vi "Flush File Data.vi"(8 "error in (no error)":errorcluster, 10 "File Log Spec in":T1={"Directory"=path "", "Groups"=[], "Buffer Size"=0, "Properties"=[], "Pretrigger"=FALSE, "Pretrigger Samples"=0, "Name"="", "Timestamp"=FALSE, "Error"=0, "Auto Open"=FALSE, "File Node Ref"=18446744073709551615, "Archive"=FALSE, "Archive Directory"=path "", "Segment Files"=FALSE, "Segment Files By"=enum."Size", "Segment Size"=100000, "Flushed Data Size Total"=0, "Append Waveform Properties"=FALSE, "Logging State"=enum."Not Started", "First Sample Start Time"=timestamp(0 s since 1904-01-01), "System dt"=0.0} {"File Node Ref" format="%.0x"}, 11 "TDMS File Ref in":refnum<k34>) -> (0 "error out":errorcluster, 2 "File Log Spec out":T1={"Directory"=path "", "Groups"=[], "Buffer Size"=0, "Properties"=[], "Pretrigger"=FALSE, "Pretrigger Samples"=0, "Name"="", "Timestamp"=FALSE, "Error"=0, "Auto Open"=FALSE, "File Node Ref"=18446744073709551615, "Archive"=FALSE, "Archive Directory"=path "", "Segment Files"=FALSE, "Segment Files By"=enum."Size", "Segment Size"=100000, "Flushed Data Size Total"=0, "Append Waveform Properties"=FALSE, "Logging State"=enum."Not Started", "First Sample Start Time"=timestamp(0 s since 1904-01-01), "System dt"=0.0} {"File Node Ref" format="%.0x"}, 3 "TDMS File Ref out":refnum<k34>)   [LabVIEW 2027, in "Embedded Data Logger Engine.lvlib"]
uses:
  Embedded Data Logger Engine.lvlib
  File Logging Specification.ctl
  Group Logging Specification.ctl
  Group Buffer Data.ctl
  Property Specification.ctl
  <vilib>/NI VeriStand/Custom Device API/Custom Device Item Ref.ctl
  Shared/Segment Files By.ctl
  Logging State.ctl
  Add to Flushed Data Size.vi
  <vilib>/NI VeriStand/Custom Device API/Custom Device API.lvlib
  Shared/Embedded Data Logger Shared.lvlib
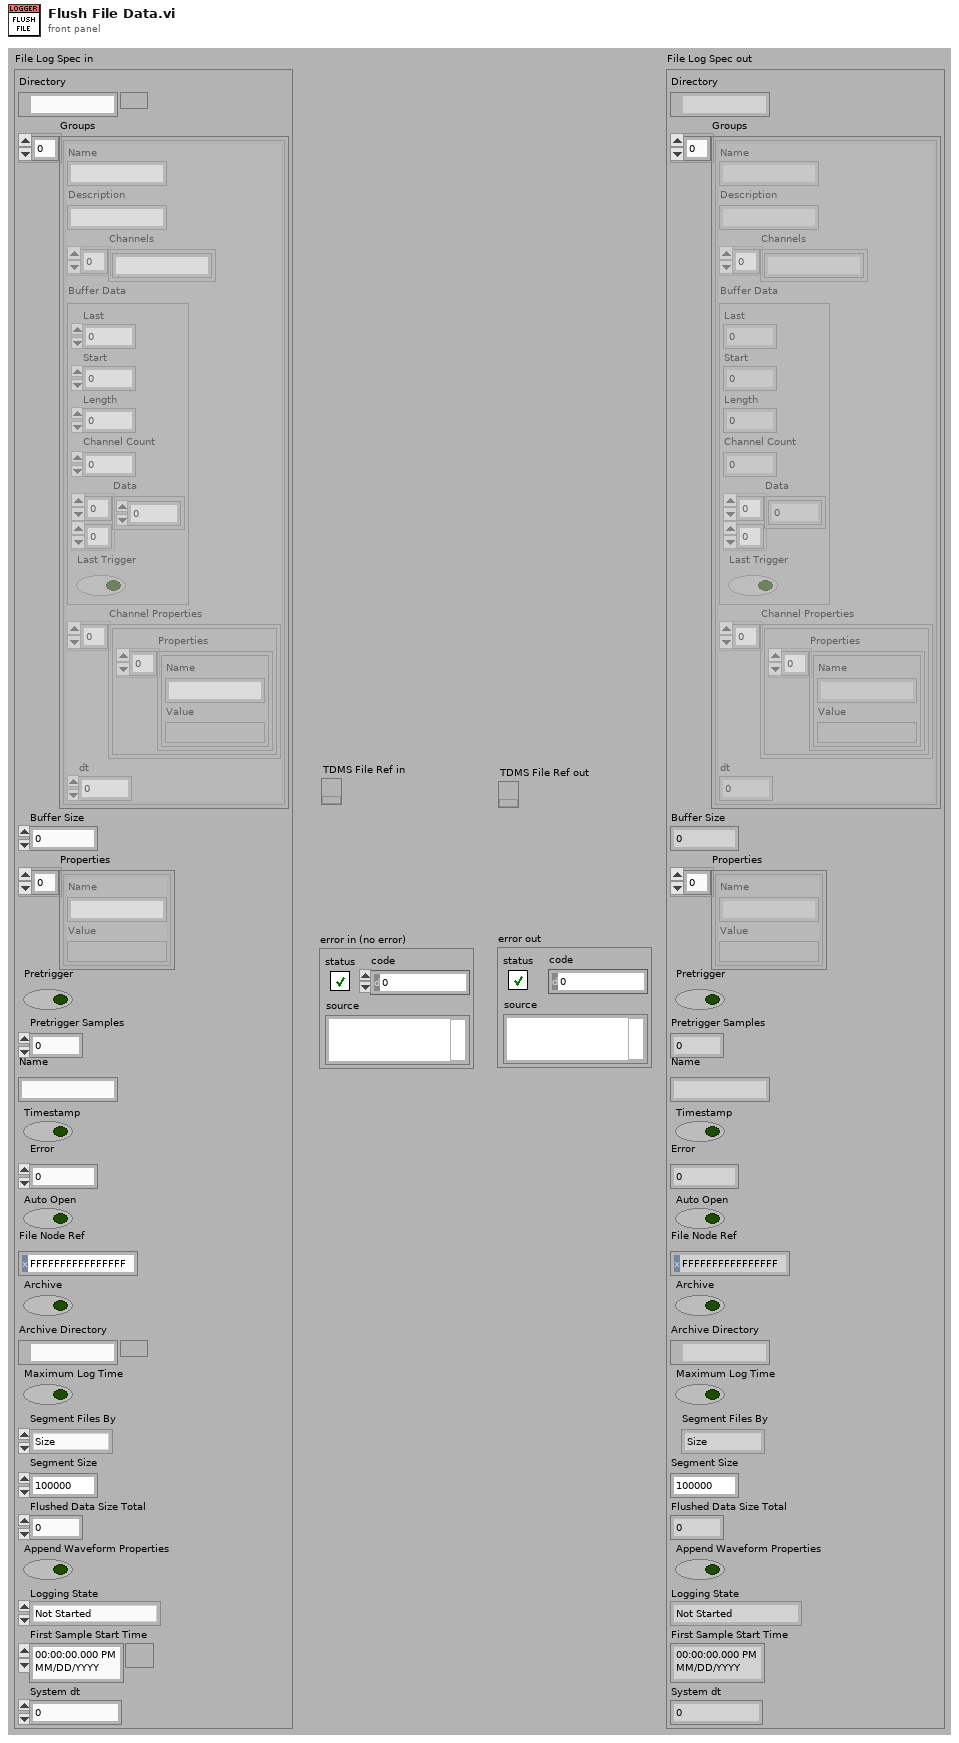
[diagram p1: front panel]
types:
  T1 = typedef "Embedded Data Logger Engine.lvlib/File Logging Specification.ctl" = cluster{"Directory":path, "Groups":T2[], "Buffer Size":i32, "Properties":T4[], "Pretrigger":bool, "Pretrigger Samples":i32, "Name":string, "Timestamp":bool, "Error":i32, "Auto Open":bool, "File Node Ref":T5, "Archive":bool, "Archive Directory":path, "Segment Files":bool, "Segment Files By":T6, "Segment Size":u32, "Flushed Data Size Total":u32, "Append Waveform Properties":bool, "Logging State":T7, "First Sample Start Time":timestamp, "System dt":dbl}
  T2 = typedef "Embedded Data Logger Engine.lvlib/Group Logging Specification.ctl" = cluster{"Name":string, "Description":string, "Channels":string[], "Buffer Data":T3, "Channel Properties":cluster{"Properties":T4[]}[], "dt":dbl}
  T3 = typedef "Embedded Data Logger Engine.lvlib/Group Buffer Data.ctl" = cluster{"Last":i32, "Start":i32, "Length":i32, "Channel Count":i32, "Data":dbl[][], "Last Trigger":bool}
  T4 = typedef "Embedded Data Logger Engine.lvlib/Property Specification.ctl" = cluster{"Name":string, "Value":variant}
  T5 = typedef "Custom Device API.lvlib/Custom Device Item Ref.ctl" = u64
  T6 = typedef "Embedded Data Logger Shared.lvlib/Segment Files By.ctl" = enum16{"Time", "Size"}
  T7 = typedef "Embedded Data Logger Engine.lvlib/Logging State.ctl" = enum16{"Not Started", "Continous Logging", "Paused", "Discontinous Logging"}
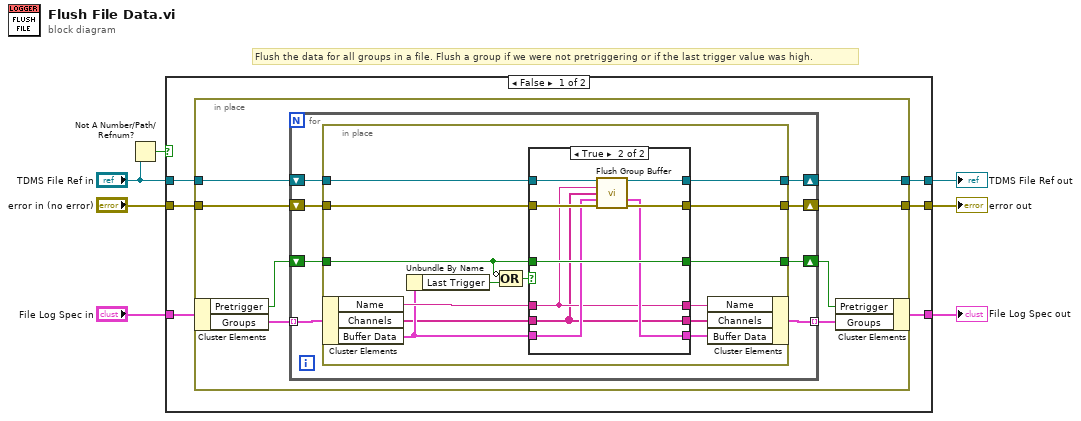
[diagram p0: block diagram]
diagram:
  # "Flush the data for all groups in a file. Flush a group if we were not pretriggering or if the last trigger value was high."
  n1 = Not A Number/Path/Refnum?(number/path/refnum="TDMS File Ref in") -> (NaN/Path/Refnum?=w1:bool)
  n2 = case shown="False" w1 {
    tunnel: "File Log Spec in" -> [w13 w59]
    tunnel: "TDMS File Ref in" -> [w12 w61]
    tunnel: [w11 w61] -> w5
    tunnel: [w10 w59] -> w7
    tunnel: "error in (no error)" -> [w9 w60]
    tunnel: [w8 w60] -> w6
    frame False {
      n3 = in-place {
        in-place-border: w12 -> [w21]
        in-place-border: [w20] -> w11
        in-place-border: w9 -> [w15]
        in-place-border: [w14] -> w8
        n4 = in-place-cluster #1(w13) -> ("Pretrigger"=w17:bool, "Groups"=w19:T2[])
        n5 = for {
          tunnel: w19 -> [w27] mode=indexing
          tunnel: [w26] -> w18 mode=indexing
          shift-right: [w28] -> w20
          shift-left: w21 -> [w29]
          shift-right: [w25] -> w16
          shift-left: w17 -> [w24]
          shift-right: [w22] -> w14
          shift-left: w15 -> [w23]
          n6 = in-place {
            in-place-border: w24 -> [w34]
            in-place-border: w29 -> [w38]
            in-place-border: [w39] -> w28
            in-place-border: [w33] -> w25
            in-place-border: w23 -> [w32]
            in-place-border: [w31] -> w22
            n7 = in-place-cluster #2(w27) -> ("Name"=w43:string, "Channels"=w30:string[], "Buffer Data"=w37:T3)
            n8 = Unbundle By Name(w37) -> ("Last Trigger"=w35:bool)
            n9 = Compound Arithmetic op=OR(invert w34, w35) -> (w36:bool)
            n10 = case shown="True" w36 {
              tunnel: w37 -> [w49 w53]
              tunnel: w43 -> [w48 w51]
              tunnel: [w49 w55] -> w42
              tunnel: w30 -> [w47 w50]
              tunnel: [w48 w51] -> w41
              tunnel: [w47 w50] -> w40
              tunnel: [w46 w52] -> w39
              tunnel: w38 -> [w46 w54]
              tunnel: [w45 w56] -> w33
              tunnel: w34 -> [w45 w56]
              tunnel: w32 -> [w44 w58]
              tunnel: [w44 w57] -> w31
              frame False {
                # "Ignore pretriggered data that hasn't already been flushed."
              }
              frame True {
                n11 = call "Flush Group Buffer.vi"("TDMS File Ref in"=w54, "Group Name"=w51, "Channels"=w50, "Group Buffer Data in"=w53, "error in (no error)"=w58) -> ("TDMS File Ref out"=w52:refnum<k34>, "Group Buffer Data out"=w55:T3, "error out"=w57:errorcluster)  [unwired: 1 in, 7 out]
              }
            }
            n12 = in-place-cluster #2("Name"=w41, "Channels"=w40, "Buffer Data"=w42) -> (w26:T2)
          }
        }
        n13 = in-place-cluster #1("Pretrigger"=w16, "Groups"=w18) -> (w10:T1)
      }
    }
    frame True {
      # "File is not open. No data to flush."
    }
  }
  "File Log Spec out" <- w7
  "error out" <- w6
  "TDMS File Ref out" <- w5
